vi "AuMT8852B Single-Slot Sensitivity Extended Results Query.vi"(7 "Stage":T1(ring), 8 "error in (no error)":errorcluster, 11 "VISA session":refnum<visa-resource-name>) -> (0 "error out":errorcluster, 2 "error code":i32, 3 "VISA session out":refnum<visa-resource-name>, 4 "Results":T2 {"Overall FER" format="%.2f"; "Overall BER" format="%.2f"})   [LabVIEW 2017]
doc: "Anritsu MT8852B Bluetooth Tester\n\nReturns the results of the Single-slot Sensitivity test.\n\nINPUTS\nStage - results of the individual hopping stages of the test.\n\nOUTPUTS\nResults - measurements made during the test."
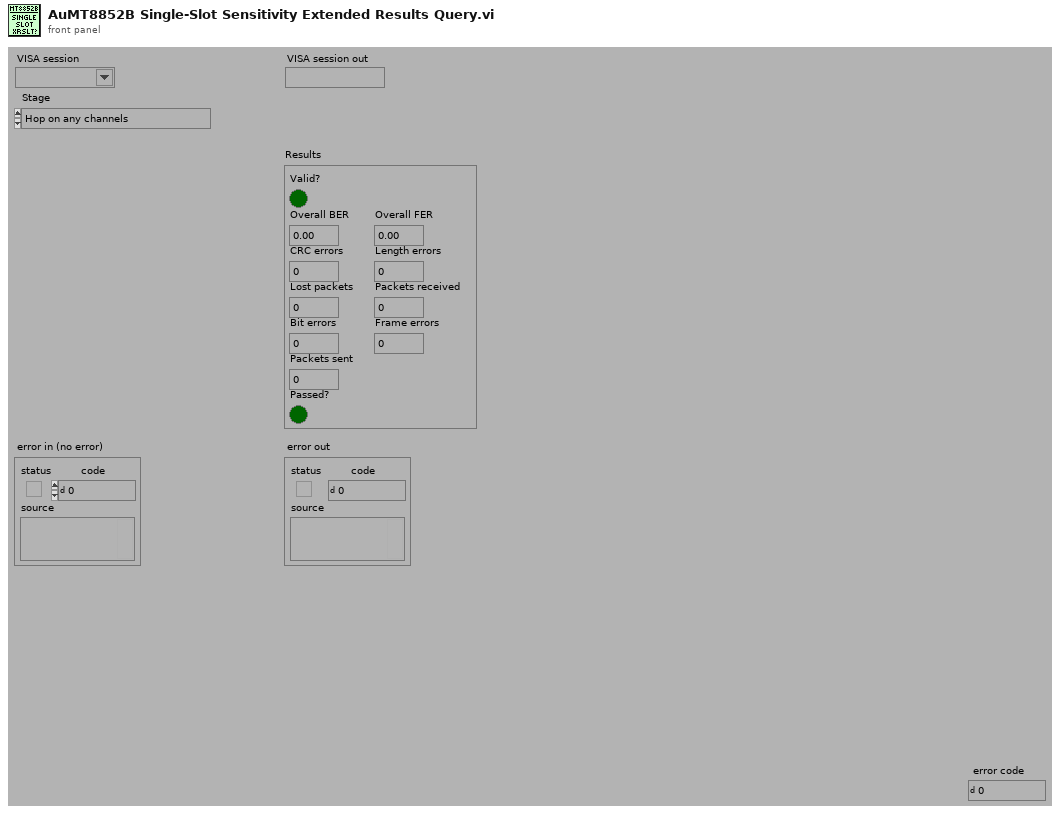
[diagram p1: front panel]
types:
  T1 = enum16{"Hop on any channels", "Hop off low frequency", "Hop off medium frequency", "Hop off high frequency"}
  T2 = cluster{"Valid?":bool, "Overall BER":dbl, "Overall FER":dbl, "CRC errors":i32, "Length errors":i32, "Lost packets":i32, "Passed?":bool, "Packets received":i32, "Bit errors":i32, "Frame errors":i32, "Packets sent":i32}
  T3 = enum16{"Simulate", "Range check", "Cache", "Query instrument status"}
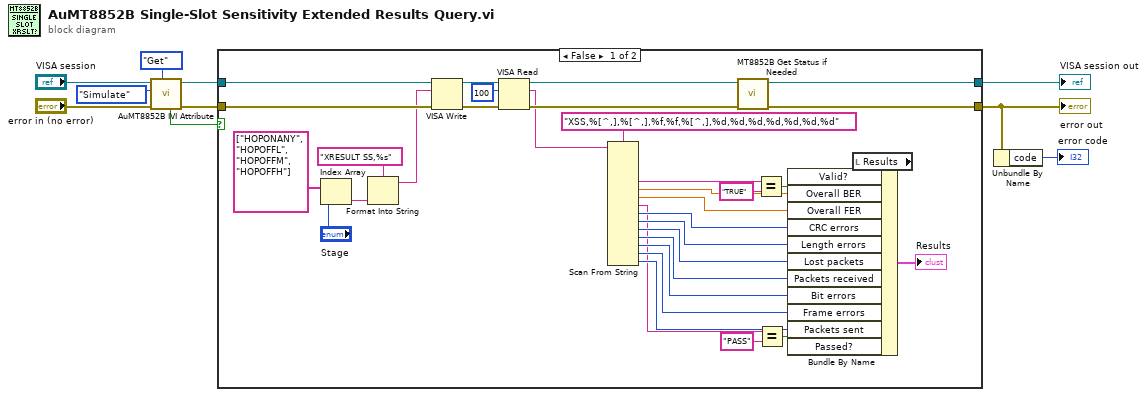
[diagram p0: block diagram]
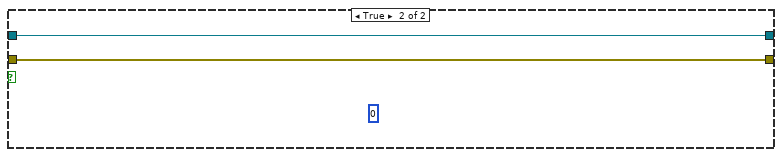
[diagram p2: hidden frame]
diagram:
  n1 = call <instrlib>:"AuMT8852B IVI Attribute.vi"("Set/Get (Set)"=enum16{"Set", "Get"}."Get", "error in (no error)"="error in (no error)", "Flag (Simulate)"=T3."Simulate", "VISA session"="VISA session") -> ("error out"=w7:errorcluster, "VISA session out"=w9:refnum<visa-resource-name>, "Value out"=w3:bool)  [unwired: 5 in]
  n2 = case shown="False" w3 {
    tunnel: [w35 w45] -> w10
    tunnel: [w34 w44] -> w1
    tunnel: w9 -> [w43 w45]
    tunnel: w7 -> [w42 w44]
    frame False {
      n3 = Index Array(array=string[] ["HOPONANY", "HOPOFFL", "HOPOFFM", "HOPOFFH"], index="Stage") -> (element=w26:string)
      n4 = Format Into String(format string="XRESULT SS,%s" ("write buffer (\"\")"), w26) -> (resulting string=w13:string)  [unwired: 2 in, 1 out]
      n5 = VISA Write(VISA resource name=w43, write buffer=w13, error in (no error)=w42) -> (VISA resource name out=w41:refnum<visa-resource-name>, error out=w40:errorcluster)  [unwired: 1 out]
      n6 = VISA Read(VISA resource name=w41, byte count=u32 100 ("byte count (0)"), error in (no error)=w40) -> (VISA resource name out=w30:refnum<visa-resource-name>, read buffer=w12:string, error out=w29:errorcluster)  [unwired: 1 out]
      n7 = Scan From String(format string="XSS,%[^,],%[^,],%f,%f,%[^,],%d,%d,%d,%d,%d,%d,%d" ("Format String"), input string=w12) -> (output 2=w24:string, output 3=w23:dbl, output 4=w22:dbl, output 5=w11:string, output 6=w21:i32, output 7=w20:i32, output 8=w19:i32, output 9=w18:i32, output 10=w17:i32, output 11=w16:i32, output 12=w15:i32)  [unwired: 15 in, 3 out]
      n8 = call <instrlib>:"MT8852B Get Status if Needed.vi"("error in (no error)"=w29, "VISA session"=w30) -> ("error out"=w34:errorcluster, "VISA session out"=w35:refnum<visa-resource-name>)  [unwired: 8 in]
      n9 = Equal?(x=w24, y="TRUE") -> (x = y?=w32:bool)
      n10 = Equal?(x=w11, y="PASS") -> (x = y?=w14:bool)
      n11 = local read "Results"() -> (w37:T2)
      n12 = Bundle By Name(cluster=w37, "Valid?"=w32, "Overall BER"=w23, "Overall FER"=w22, "CRC errors"=w21, "Length errors"=w20, "Lost packets"=w19, "Packets received"=w18, "Bit errors"=w17, "Frame errors"=w16, "Packets sent"=w15, "Passed?"=w14) -> (→"Results":T2)
    }
    frame True {
      (unwired) u8 0
    }
  }
  "error out" <- w1
  "VISA session out" <- w10
  n13 = Unbundle By Name(w1) -> ("code"=→"error code":i32)
